vi "R2R-Controller.vi"(4 "Custom Controller Inputs":T1, 6 "Gain Configuration":T2={"PID Gains"={"proportional gain (Kc)"=1.0, "integral gain (Kc*Ts/Ti)"=0.0, "derivative gain (Kc*Td/Ts)"=0.0}, "Output Range"={"output high"=10.0, "output low"=-10.0}}, 7 "Reset Integrator":bool, 8 "X (Raw Analog V)":fxp<+,18,3>, 9 "F (Raw Analog V)":fxp<+,18,3>, 10 "X* (mm)":fxp<+/-,16,7>, 11 "F* (N)":fxp<+/-,16,7>) -> (0 "Xmeas (mm)":fxp<+,30,7>, 1 "Fmeas (N)":fxp<+/-,40,11>, 2 "V*(V)":fxp<+/-,53,13> format="%.6f", 3 "PWM Duty Cycle":i16, 5 "Duty Cycle Output":i16)   [LabVIEW 2013]
uses:
  controls/Control Configuration.ctl
  controls/Custom Controller Inputs.ctl
  <vilib>/rvi/Analysis/measure/butterworth/XNode/niFpgaButterworthFilter.xnode
  <vilib>/addons/control/pid/fpga.llb/XNode/niFpgaPID.xnode
panel:
  out "Y*'":fxp<+/-,36,31>
  out "Y*":fxp<+/-,64,27> format="%.41g"
  in  "K_PosSense (mm/Volt)":fxp<+,12,4>=10.0
  out "deltaX*":fxp<+/-,49,21> format="%.34g"
  out "Ferr (N)":fxp<+/-,40,11>
  in  "K_PWM (Counts/Volt)":fxp<+,16,7>=83.33203125
  in  "Ra (Armature Resistance) (Ohms)":fxp<+/-,7,7>=60.0
  out "I* Current Command (A)":fxp<+/-,48,8>
  in  "Force Sensor Gain (N/V)":fxp<+,20,6>=53.02703857421875
  in  "L12 Gain (mA/N)":fxp<+,16,2>=2.29180908203125
  in  "L12 Offset (mA)":fxp<+,18,4>=12.9949951171875
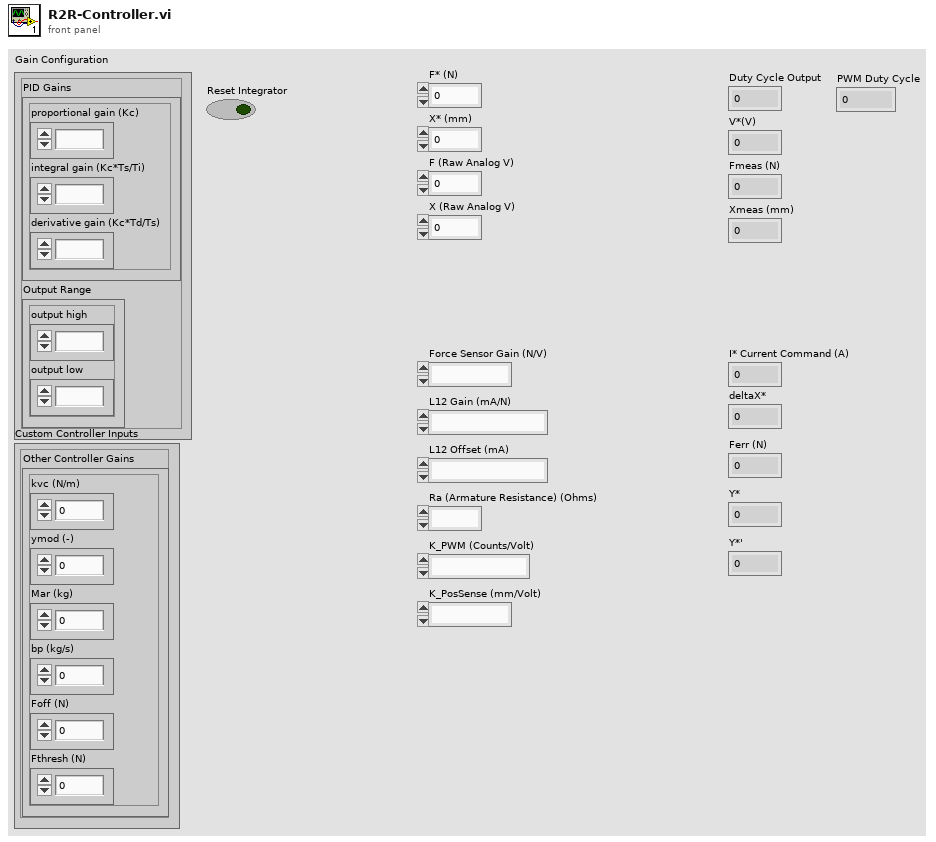
[diagram p1: front panel]
types:
  T1 = typedef "Custom Controller Inputs.ctl" = cluster{"Other Controller Gains":cluster{"kvc (N/m)":fxp<+,16,12>, "ymod (-)":fxp<+/-,16,5>, "Mar (kg)":fxp<+/-,16,8>, "bp (kg/s)":fxp<+/-,16,5>, "Foff (N)":fxp<+/-,16,8>, "Fthresh (N)":fxp<+/-,16,5>}}
  T2 = typedef "Control Configuration.ctl" = cluster{"PID Gains":cluster{"proportional gain (Kc)":fxp<+/-,16,8>, "integral gain (Kc*Ts/Ti)":fxp<+/-,16,8>, "derivative gain (Kc*Td/Ts)":fxp<+/-,16,8>}, "Output Range":cluster{"output high":fxp<+/-,16,7>, "output low":fxp<+/-,16,7>}}
  T3 = cluster{"kvc (N/m)":fxp<+,16,12>, "ymod (-)":fxp<+/-,16,5>, "Mar (kg)":fxp<+/-,16,8>, "bp (kg/s)":fxp<+/-,16,5>, "Foff (N)":fxp<+/-,16,8>, "Fthresh (N)":fxp<+/-,16,5>}
  T4 = cluster{"proportional gain (Kc)":fxp<+/-,16,8>, "integral gain (Kc*Ts/Ti)":fxp<+/-,16,8>, "derivative gain (Kc*Td/Ts)":fxp<+/-,16,8>}
  T5 = cluster{"output high":fxp<+/-,16,7>, "output low":fxp<+/-,16,7>}
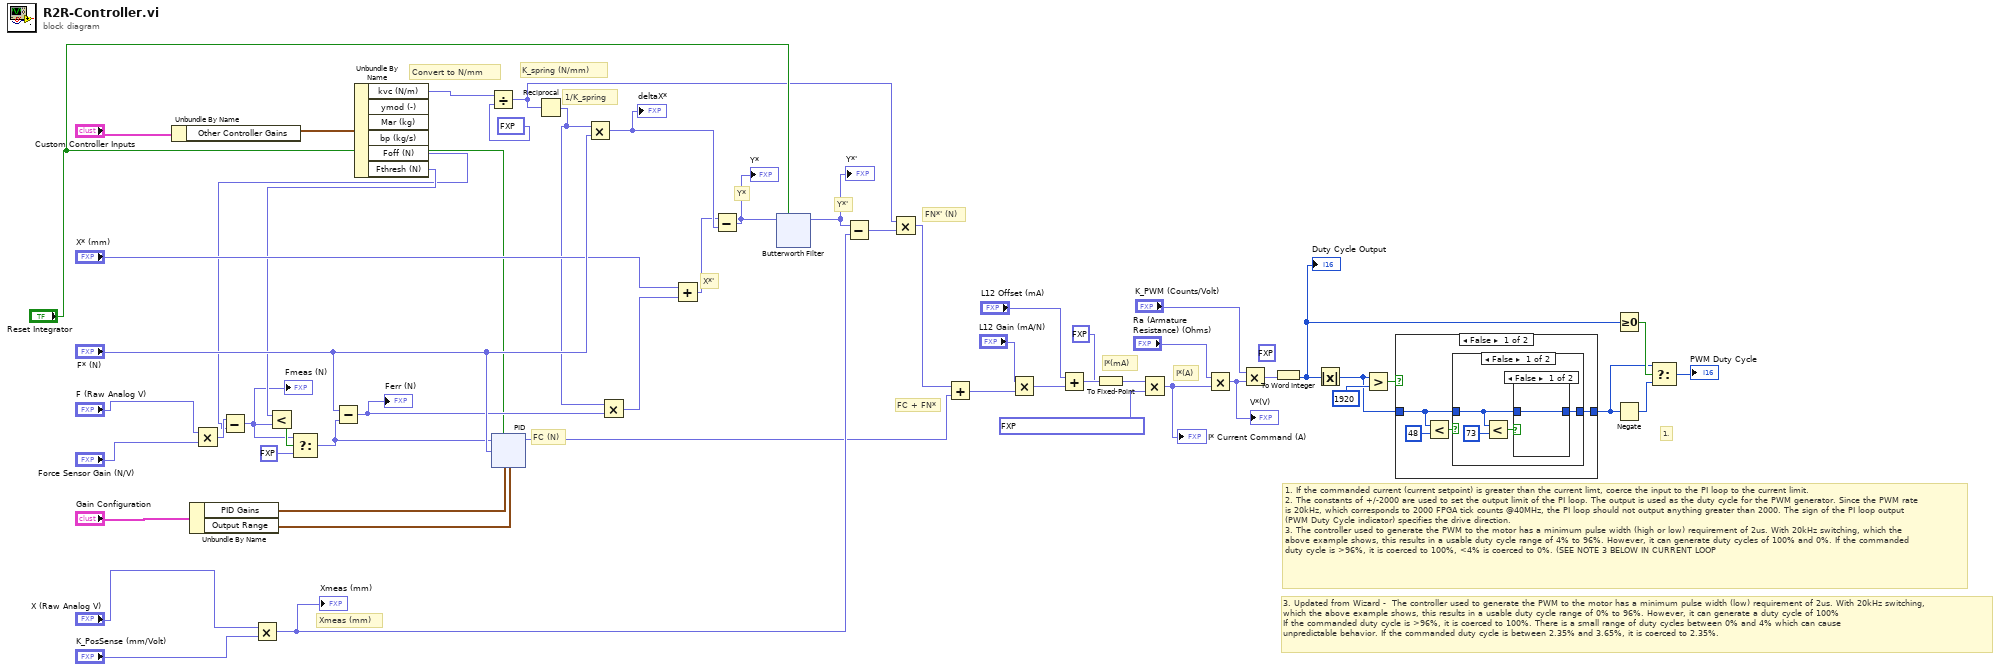
[diagram p0: block diagram]
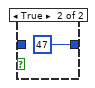
[diagram p2: hidden frame]
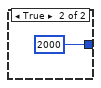
[diagram p4: hidden frame]
diagram:
  (unwired) fxp<+/-,16,16> 0.0 ("fixed-point type")
  # "FC + FN*"
  # "K_spring (N/mm)"
  # "Convert to N/mm"
  # "1. If the commanded current (current setpoint) is greater than the current limt, coerce the input to the PI loop to the current limit.\n2. The constants of +/-2000 are used to set the output limit of the PI loop. The output is used as the duty cycle for the PWM generator. Since the PWM rate is 20kHz, which corresponds to 2000 FPGA tick counts @40MHz, the PI loop should not output anything greater than 2000. The sign of the PI loop output (PWM Duty Cycle indicator) specifies the drive direction.\n3. The controller used to generate the PWM to the motor has a minimum pulse width (high or low) requirement of 2us. With 20kHz switching, which the above example shows, this results in a usable duty cycle range of 4% to 96%. However, it can generate duty cycles of 100% and 0%. If the commanded duty cycle is >96%, it is coerced to 100%, <4% is coerced to 0%. (SEE NOTE 3 BELOW IN CURRENT LOOP"
  # "3. Updated from Wizard -  The controller used to generate the PWM to the motor has a minimum pulse width (low) requirement of 2us. With 20kHz switching, which the above example shows, this results in a usable duty cycle range of 0% to 96%. However, it can generate a duty cycle of 100%\nIf the commanded duty cycle is >96%, it is coerced to 100%. There is a small range of duty cycles between 0% and 4% which can cause\nunpredictable behavior. If the commanded duty cycle is between 2.35% and 3.65%, it is coerced to 2.35%."
  # "1."
  # "Y*'"
  # "I*(A)"
  # "I*(mA)"
  # "FC (N)"
  # "FN*' (N)"
  # "Xmeas (mm)"
  # "Y*"
  # "X*'"
  # "1/K_spring"
  n1 = Unbundle By Name("Custom Controller Inputs") -> ("Other Controller Gains"=w49:T3)
  n2 = Unbundle By Name("Gain Configuration") -> ("PID Gains"=w53:T4, "Output Range"=w52:T5)
  n3 = Multiply(x="F (Raw Analog V)", y="Force Sensor Gain (N/V)") -> (x*y=w10:fxp<+,38,9>)
  n4 = Multiply(x="X (Raw Analog V)", y="K_PosSense (mm/Volt)") -> (x*y=w41:fxp<+,30,7>)
  "Xmeas (mm)" <- w41
  n5 = Unbundle By Name(w49) -> ("kvc (N/m)"=w1:fxp<+,16,12>, "Foff (N)"=w9:fxp<+/-,16,8>, "Fthresh (N)"=w11:fxp<+/-,16,5>)  [unwired: 3 out]
  n6 = Subtract(x=w10, y=w9) -> (x-y=w8:fxp<+/-,40,11>)
  "Fmeas (N)" <- w8
  n7 = Less?(x=w11, y=w8) -> (x < y?=w17:bool)
  n8 = Select(t=w8, s=w17, f=fxp<+,38,9> 0.0) -> (s? t:f=w15:fxp<+/-,40,11>)
  n9 = Subtract(x="F* (N)", y=w15) -> (x-y=w47:fxp<+/-,40,11>)
  "Ferr (N)" <- w47
  n10 = Divide(x=w1, y=fxp<+,17,10> 1000.0) -> (x/y=w5:fxp<+,33,19>)
  n11 = xnode "PID"("process variable"=w15, "reset?"="Reset Integrator", "setpoint"="F* (N)", "PID gains"=w53, "output range"=w52) -> ("output"=w38:fxp<+/-,16,11>)
  n12 = Reciprocal(x=w5) -> (1/x=w6:fxp<+,34,15>)
  n13 = Multiply(x=w6, y="F* (N)") -> (x*y=w44:fxp<+/-,49,21>)
  "deltaX*" <- w44
  n14 = Multiply(x=w6, y=w47) -> (x*y=w45:fxp<+/-,64,25>)
  n15 = Add(x="X* (mm)", y=w45) -> (x+y=w43:fxp<+/-,64,26>)
  n16 = Subtract(x=w43, y=w44) -> (x-y=w29:fxp<+/-,64,27>)
  "Y*" <- w29
  n17 = xnode "Butterworth Filter"("input data"=w29, "reset"="Reset Integrator") -> ("output data"=w28:fxp<+/-,36,31>)  [unwired: 1 in]
  "Y*'" <- w28
  n18 = Subtract(x=w28, y=w41) -> (x-y=w40:fxp<+/-,55,32>)
  n19 = Multiply(x=w5, y=w40) -> (x*y=w39:fxp<+/-,64,50>)
  n20 = Add(x=w39, y=w38) -> (x+y=w36:fxp<+/-,64,51>)
  n21 = Multiply(x="L12 Gain (mA/N)", y=w36) -> (x*y=w35:fxp<+/-,64,53>)
  n22 = Add(x="L12 Offset (mA)", y=w35) -> (x+y=w20:fxp<+/-,64,54>)
  n23 = To Fixed-Point(fixed-point type=fxp<+/-,32,16> 0.0, number=w20) -> (fixed-point=w18:fxp<+/-,32,16>)
  n24 = Multiply(x=w18, y=fxp<+/-,16,-8> 0.0009999871253967285) -> (x*y=w12:fxp<+/-,48,8>)
  "I* Current Command (A)" <- w12
  n25 = Multiply(x="Ra (Armature Resistance) (Ohms)", y=w12) -> (x*y=w31:fxp<+/-,53,13>)
  "V*(V)" <- w31
  n26 = Multiply(x="K_PWM (Counts/Volt)", y=w31) -> (x*y=w14:fxp<+/-,64,20>)
  n27 = To Word Integer(number=w14) -> (16bit integer=w13:i16)
  "Duty Cycle Output" <- w13
  n28 = Absolute Value(x=w13) -> (abs(x)=w22:i16)
  n29 = Greater?(x=w22, y=i16 1920 ("upper limit")) -> (0:w24:bool)
  n30 = case shown="False" w24 {
    tunnel: [w57 i16 2000 ("upper limit")] -> w23
    tunnel: w22 -> [w55 _]
    frame False {
      n31 = Less?(x=w55, y=i16 48 ("lower limit")) -> (x < y?=w56:bool)
      n32 = case shown="False" w56 {
        tunnel: [w59 w65] -> w57
        tunnel: w55 -> [w60 w65]
        frame False {
          n33 = Less?(x=w60, y=i16 73 ("lower limit")) -> (x < y?=w61:bool)
          n34 = case shown="False" w61 {
            tunnel: w60 -> [w63 _]
            tunnel: [w63 i16 47 ("lower limit")] -> w59
            frame False {
            }
            frame True {
            }
          }
        }
        frame True {
        }
      }
    }
    frame True {
    }
  }
  n35 = Greater Or Equal To 0?(x=w13) -> (x >= 0?=w27:bool)
  n36 = Negate(x=w23) -> (-x=w26:i16)
  n37 = Select(t=w23, s=w27, f=w26) -> (s? t:f=→"PWM Duty Cycle":i16)
